vi "Trim Whitespace One-Sided.vi"(0 "string":string, 1 "reverse?":bool, 2 "enable?":bool) -> (3 "trimmed string":string)   [LabVIEW 2024]
doc: "Conditionally trim whitespace from either the beginning or the end of <b>string</b>."
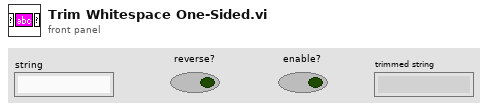
[diagram p1: front panel]
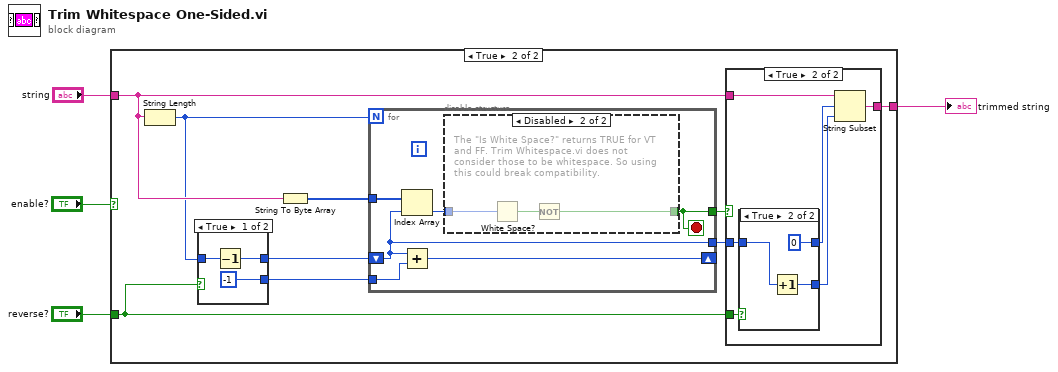
[diagram p0: block diagram]
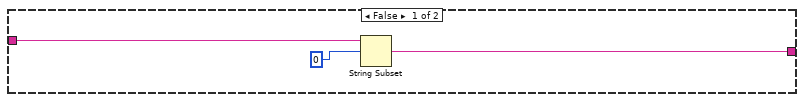
[diagram p2: hidden frame]
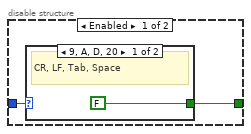
[diagram p3: hidden frame]
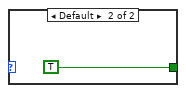
[diagram p4: hidden frame]
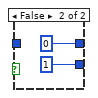
[diagram p5: hidden frame]
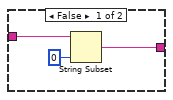
[diagram p6: hidden frame]
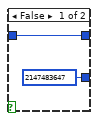
[diagram p7: hidden frame]
diagram:
  n1 = case shown="True" "enable?" {
    tunnel: "string" -> [w6 w16]
    tunnel: [w5 w15] -> w3
    tunnel: "reverse?" -> [_ w9]
    frame False {
      n2 = String Subset(string=w6, offset (0)=0) -> (substring=w5:string)  [unwired: 1 in]
    }
    frame True {
      n3 = String Length(string=w16) -> (length=w14:i32)
      n4 = case shown="True" w9 {
        tunnel: w14 -> [w31 _]
        tunnel: [w30 0] -> w13
        tunnel: [-1 ("length (rest)") 1 ("length (rest)")] -> w11
        frame True {
          n5 = Decrement(x=w31) -> (x-1=w30:i32)
        }
        frame False {
        }
      }
      n6 = String To Byte Array(string=w16) -> (unsigned byte array=w10:u8[])
      n7 = for {
        N: w14 -> [_]
        tunnel: w10 -> [w22]
        tunnel: [w20] -> w12
        shift-right: [w19] -> _
        shift-left: w13 -> [w17]
        tunnel: w11 -> [w18]
        tunnel: [w17] -> w8
        stop <- w20 stop-if-true
        n8 = Index Array(array=w22, index=w17) -> (element=w21:u8)
        n9 = Add(x=w17, y=w18) -> (x+y=w19:i32)
        n10 = disable-structure shown="Disabled" {
          disable-tunnel: w21 -> [w24 w29]
          disable-tunnel: [w23 w27] -> w20
          frame Enabled {
            n11 = case shown="9, A, D, 20" w24 {
              tunnel: [FALSE TRUE] -> w23
              frame 9, 10, 13, 32 {
                # "CR, LF, Tab, Space"
              }
              frame Default {
              }
            }
          }
          frame Disabled {
            # "The \"Is White Space?\" returns TRUE for VT and FF. Trim Whitespace.vi does not consider those to be whitespace. So using this could break compatibility."
            n12 = White Space?(1:w29) -> (0:w28:bool)
            n13 = Not(x=w28) -> (.not. x?=w27:bool)
          }
        }
      }
      n14 = case shown="True" w12 {
        tunnel: w16 -> [w37 w43]
        tunnel: [w36 w42] -> w15
        tunnel: w9 -> [_ w41]
        tunnel: w8 -> [_ w40]
        frame False {
          n15 = String Subset(string=w37, length (rest)=0 ("length (rest)")) -> (substring=w36:string)  [unwired: 1 in]
        }
        frame True {
          n16 = case shown="True" w41 {
            tunnel: w40 -> [w44 w47]
            tunnel: [w44 0] -> w39
            tunnel: [2147483647 w46] -> w38
            frame False {
            }
            frame True {
              n17 = Increment(x=w47) -> (x+1=w46:i32)
            }
          }
          n18 = String Subset(string=w43, offset (0)=w39, length (rest)=w38) -> (substring=w42:string)
        }
      }
    }
  }
  "trimmed string" <- w3
